vi "AT.vi"(6 "时间值":i32, 8 "数值":i16, 9 "width":i32[](array[numeric]), 10 "begin":i32[](array[numeric]), 11 "act":bool[](array[boolean])) -> (2 "添加的数组":bool[](array[boolean]))   [LabVIEW 2018]
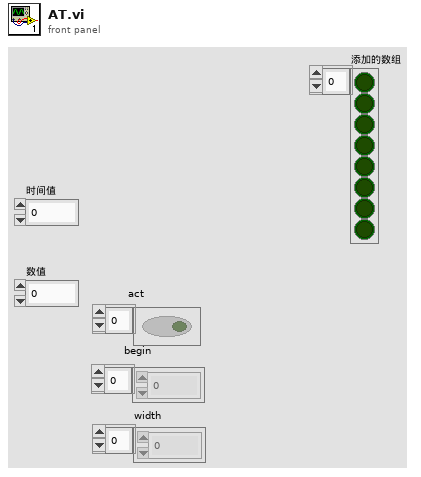
[diagram p1: front panel]
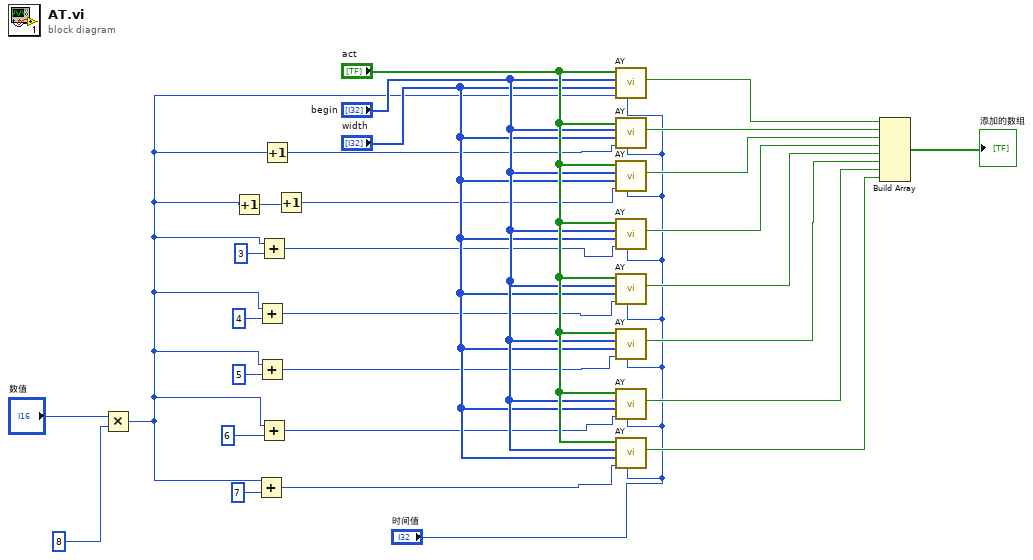
[diagram p0: block diagram]
diagram:
  n1 = Multiply(x="数值", y=i16 8) -> (x*y=w5:i16)
  n2 = Increment(x=w5) -> (x+1=w13:i16)
  n3 = Add(x=w5, y=i16 7) -> (x+y=w1:i16)
  n4 = Add(x=w5, y=i16 4) -> (x+y=w4:i16)
  n5 = Add(x=w5, y=i16 5) -> (x+y=w3:i16)
  n6 = Add(x=w5, y=i16 3) -> (x+y=w10:i16)
  n7 = Add(x=w5, y=i16 6) -> (x+y=w2:i16)
  n8 = Increment(x=w5) -> (x+1=w14:i16)
  n9 = Increment(x=w13) -> (x+1=w12:i16)
  n10 = call "AY.vi"("时间值"="时间值", "数值"=w5, "width"="width", "begin"="begin", "act"="act") -> ("布尔"=w26:bool)  [unwired: 6 in]
  n11 = call "AY.vi"("时间值"="时间值", "数值"=w14, "width"="width", "begin"="begin", "act"="act") -> ("布尔"=w25:bool)  [unwired: 6 in]
  n12 = call "AY.vi"("时间值"="时间值", "数值"=w12, "width"="width", "begin"="begin", "act"="act") -> ("布尔"=w24:bool)  [unwired: 6 in]
  n13 = call "AY.vi"("时间值"="时间值", "数值"=w10, "width"="width", "begin"="begin", "act"="act") -> ("布尔"=w23:bool)  [unwired: 6 in]
  n14 = call "AY.vi"("时间值"="时间值", "数值"=w4, "width"="width", "begin"="begin", "act"="act") -> ("布尔"=w22:bool)  [unwired: 6 in]
  n15 = call "AY.vi"("时间值"="时间值", "数值"=w3, "width"="width", "begin"="begin", "act"="act") -> ("布尔"=w21:bool)  [unwired: 6 in]
  n16 = call "AY.vi"("时间值"="时间值", "数值"=w2, "width"="width", "begin"="begin", "act"="act") -> ("布尔"=w20:bool)  [unwired: 6 in]
  n17 = call "AY.vi"("时间值"="时间值", "数值"=w1, "width"="width", "begin"="begin", "act"="act") -> ("布尔"=w19:bool)  [unwired: 6 in]
  n18 = Build Array(w26, w25, w24, w23, w22, w21, w20, w19) -> (→"添加的数组":bool[])
